vi "Receive Message.vi"(8 "error in (no error)":errorcluster, 9 "timeout ms (-1)":i32=-1, 11 "Network Stream in":refnum<class "Network Stream.lvclass">) -> (0 "error out":errorcluster, 1 "Timed out?":bool, 2 "Message":refnum<class "Message.lvclass">, 3 "Network Stream out":refnum<class "Network Stream.lvclass">, 4 "priority":i32)   [LabVIEW 2023, in "Network Stream.lvclass"]
uses:
  Network Stream.lvclass
  C:/Program Files/National Instruments/LabVIEW 2023/vi.lib/ni/Actors/Network Endpoint Actors/Abstract Classes/Message Stream/Message Stream.lvclass
  <vilib>/ActorFramework/Message/Message.lvclass
  <vilib>/ni/Actors/Network Endpoint Actors/Abstract Classes/Message Stream/Message Stream.lvclass/Message Stream.ctl
  Network Stream.lvclass/Network Stream.ctl
  <vilib>/ni/Actors/Network Endpoint Actors/Abstract Classes/Cipher/Cipher.lvclass
  <vilib>/ni/Actors/Network Endpoint Actors/Abstract Classes/Message Stream/Message Stream.lvclass
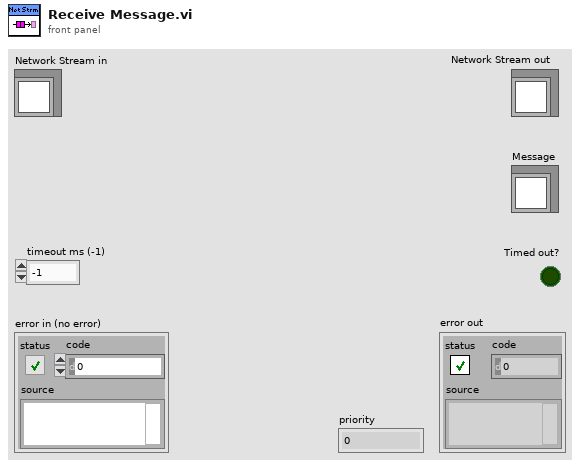
[diagram p1: front panel]
types:
  T1 = cluster{"Actor Framework.lvlib:Message.lvclass":refnum<class "Message.lvclass">, "priority":i32}
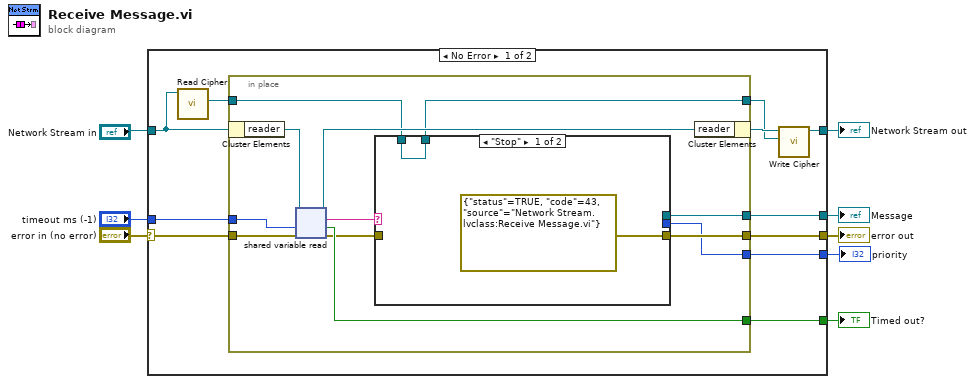
[diagram p0: block diagram]
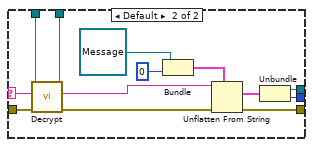
[diagram p2: hidden frame]
diagram:
  n1 = case shown="No Error" "error in (no error)" {
    selector: "error in (no error)" -> [w19 w47]
    tunnel: "Network Stream in" -> [w13 w48]
    tunnel: [w18 w47] -> w7
    tunnel: [w10 w48] -> w1
    tunnel: [w17 _] -> w6
    tunnel: [w16 _] -> w5
    tunnel: "timeout ms (-1)" -> [w15 _]
    tunnel: [w14 _] -> w3
    frame No Error {
      n2 = call <vilib>:"Read Cipher.vi"("Message Stream in"=w13) -> ("Cipher.lvclass"=w12:refnum<class "Cipher.lvclass">)  [unwired: 10 in]
      n3 = in-place {
        in-place-border: w19 -> [w29]
        in-place-border: [w28] -> w18
        in-place-border: [w27] -> w17
        in-place-border: [w26] -> w16
        in-place-border: w15 -> [w25]
        in-place-border: [w24] -> w14
        in-place-border: w12 -> [w21]
        in-place-border: [w20] -> w9
        n4 = in-place-cluster #1(w13) -> ("reader"=w31:refnum<k21>)
        n5 = shared-variable-read(w31, w29, w25) -> (w30:refnum<k21>, w22:errorcluster, w26:bool, w23:string)
        n6 = case shown="\"Stop\"" w23 {
          selector: w23 -> [_ w38]
          tunnel: w22 -> [_ w39]
          tunnel: [errorcluster {"status"=TRUE, "code"=43, "source"="Network Stream.lvclass:Receive Message.vi"} ("error out") w46] -> w28
          tunnel: [_ w41] -> w27
          tunnel: [_ w40] -> w24
          tunnel: w21 -> [w32 w35]
          tunnel: [w32 w34] -> w20
          frame "Stop" {
          }
          frame Default {
            n7 = call-dynamic "Decrypt.vi"("error in (no error)"=w39, "Ciphertext"=w38, "Cipher in"=w35) -> ("error out"=w37:errorcluster, "Plaintext"=w36:string, "Cipher out"=w34:refnum<class "Cipher.lvclass">)  [unwired: 6 in]
            n8 = Bundle("Actor Framework.lvlib:Message.lvclass"=refnum<class "Message.lvclass"> refnum, "priority"=0) -> (w42:T1)  [unwired: 1 in]
            n9 = Unflatten From String(type=w42, binary string=w36, error in (no error)=w37) -> (value=w45:T1, error out=w46:errorcluster)  [unwired: 2 in, 1 out]
            n10 = Unbundle(w45) -> ("Actor Framework.lvlib:Message.lvclass"=w41:refnum<class "Message.lvclass">, "priority"=w40:i32)
          }
        }
        n11 = in-place-cluster #1("reader"=w30) -> (w11:refnum<class "Network Stream.lvclass">)
      }
      n12 = call <vilib>:"Write Cipher.vi"("Cipher"=w9, "Message Stream in"=w11) -> ("Message Stream out"=w10:refnum<class "Network Stream.lvclass">)  [unwired: 9 in]
    }
    frame Error {
    }
  }
  "Timed out?" <- w5
  "error out" <- w7
  "Network Stream out" <- w1
  "Message" <- w6
  "priority" <- w3
